vi "4.-Nodos de Propiedades.vi"() -> ()   [LabVIEW 2020]
panel:
  in  "Boolean":bool
  in  "String":string
  in  "Deshabilitar":bool
  in  "Posicion vertical del tanque":i32(slide) scale=0.0..1000.0
  in  "Posicion horizontal del tanque":i32(slide) scale=0.0..1000.0
  in  "Limite":dbl
  out "Tanque":dbl(slide) scale=0.0..10.0
  in  "stop":bool
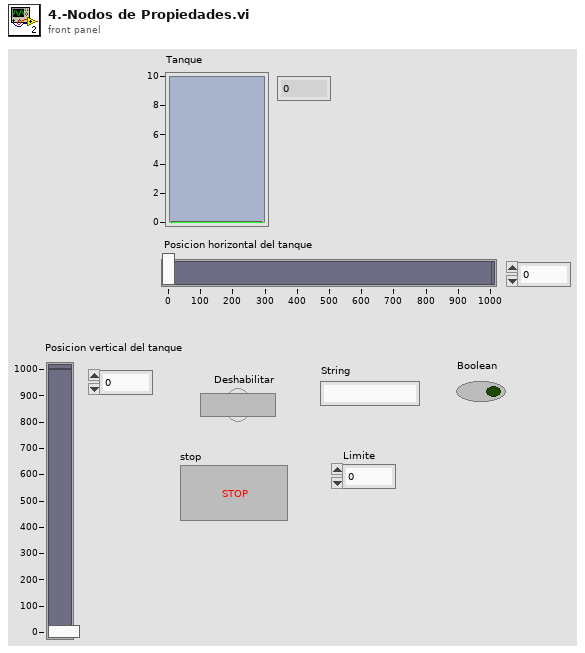
[diagram p1: front panel]
types:
  T1 = cluster{"Posicion horizontal del tanque":i32, "Posicion vertical del tanque":i32}
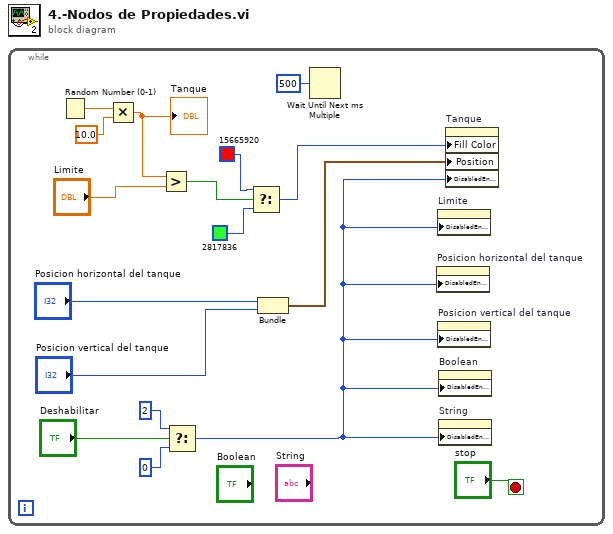
[diagram p0: block diagram]
diagram:
  n1 = while {
    stop <- "stop" stop-if-true
    n2 = Random Number (0-1)() -> (number: 0 to 1=w16:dbl)
    n3 = Multiply(x=w16, y=10.0) -> (x*y=w13:dbl)
    "Tanque" <- w13
    n4 = Greater?(x=w13, y="Limite") -> (0:w11:bool)
    n5 = Select(t=i8 2, s="Deshabilitar", f=i8 0) -> (s? t:f=w1:i8)
    n6 = Select(t=u32 15665920, s=w11, f=u32 2817836) -> (s? t:f=w8:u32)
    n7 = Bundle "Bundle"("Posicion horizontal del tanque"="Posicion horizontal del tanque", "Posicion vertical del tanque"="Posicion vertical del tanque") -> (w5:T1)  [unwired: 1 in]
    n8 = Wait Until Next ms Multiple(millisecond multiple=u32 500) -> ()  [unwired: 1 out]
    n9 = property on="Posicion horizontal del tanque" class="Slide (strict)"("DisabledEnum"=w1) -> ()  [unwired: 2 in, 2 out]
    n10 = property on="Limite" class="DigNum (strict)"("DisabledEnum"=w1) -> ()  [unwired: 2 in, 2 out]
    n11 = property on="Posicion vertical del tanque" class="Slide (strict)"("DisabledEnum"=w1) -> ()  [unwired: 2 in, 2 out]
    n12 = property on="Boolean" class="Bool (strict)"("DisabledEnum"=w1) -> ()  [unwired: 2 in, 2 out]
    n13 = property on="String" class="Str"("DisabledEnum"=w1) -> ()  [unwired: 2 in, 2 out]
    n14 = property on="Tanque" class="Slide (strict)"("Fill Color"=w8, "Position"=w5, "DisabledEnum"=w1) -> ()  [unwired: 2 in, 2 out]
  }
